vi "Get Default Values.vi"(8 "error in (no error)":errorcluster, 10 "App Config":path, 11 "Step in":refnum<class "Step.lvclass">) -> (0 "error out":errorcluster, 3 "Step out":refnum<class "Step.lvclass">)   [LabVIEW 2020, in "MacroAssert.lvlib" / "Step.lvclass"]
uses:
  Step.lvclass
  Step.lvclass/Step.ctl
  <vilib>/Utility/config.llb/NI_LVConfig.lvlib
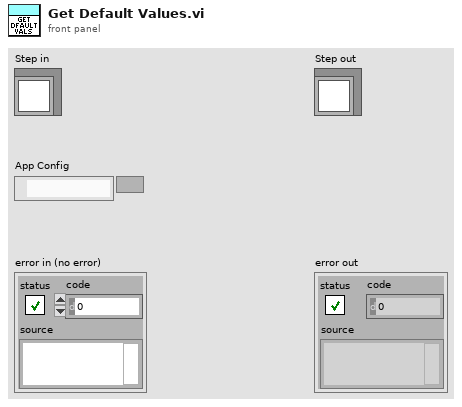
[diagram p1: front panel]
types:
  T1 = typedef "MacroAssert.lvlib/Step Type V3.ctl" = enum16{"Mouse Action", "Keyboard Action", "Window Action", "Timing Action", "Boolean Assertion", "Numeric Assertion", "String Assertion", "Image Assertion"}
  T2 = typedef "NI_LVConfig.lvlib/Config Data RefNum.ctl" = refnum<k1>
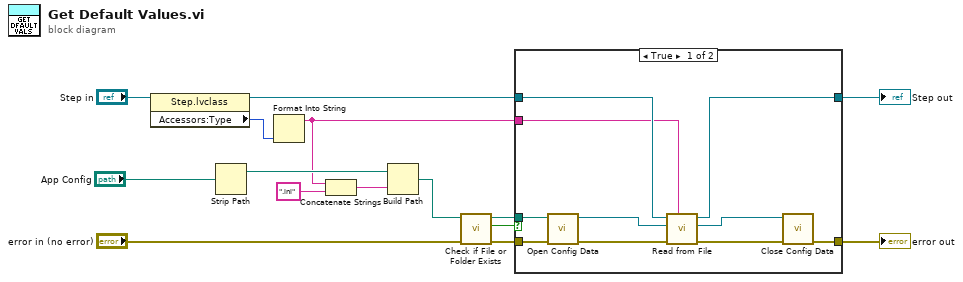
[diagram p0: block diagram]
diagram:
  n1 = property class="Step.lvclass"(reference="Step in") -> (reference out=w12:refnum<class "Step.lvclass">, "Accessors:Type"=w9:T1)  [unwired: 1 in, 1 out]
  n2 = Strip Path(path="App Config") -> (stripped path=w10:path)  [unwired: 1 out]
  n3 = Format Into String(w9) -> (resulting string=w1:string)  [unwired: 3 in, 1 out]
  n4 = Concatenate Strings(w1, ".ini" ("format string")) -> (w3:string)
  n5 = Build Path(base path=w10, name or relative path=w3) -> (appended path=w7:path)
  n6 = call <vilib>:"Check if File or Folder Exists.vi"("error in (no error)"="error in (no error)", "path"=w7) -> ("error out"=w6:errorcluster, "file or folder exists?"=w4:bool, "dup path"=w5:path)  [unwired: 7 in]
  n7 = case shown="True" w4 {
    tunnel: [w18 w27] -> w15
    tunnel: [w24 w26] -> w13
    tunnel: w12 -> [w25 w26]
    tunnel: w5 -> [w21 _]
    tunnel: w6 -> [w22 w27]
    tunnel: w1 -> [w23 _]
    frame True {
      n8 = call <vilib>:"Open Config Data.vi"("error in (no error)"=w22, "configuration file path"=w21) -> ("error out"=w20:errorcluster, "refnum"=w17:T2)  [unwired: 7 in, 1 out]
      n9 = call-dynamic "Read from File.vi"("Section Name"=w23, "error in (no error)"=w20, "INI Ref"=w17, "Step in"=w25) -> ("error out"=w19:errorcluster, "INI Ref out"=w16:T2, "Step out"=w24:refnum<class "Step.lvclass">)  [unwired: 5 in]
      n10 = call <vilib>:"Close Config Data.vi"("error in (no error)"=w19, "refnum"=w16) -> ("error out"=w18:errorcluster)  [unwired: 8 in, 1 out]
    }
    frame False {
    }
  }
  "error out" <- w15
  "Step out" <- w13
